vi "AutonTurning.vi"(7 "Re-Init":bool, 9 "SensorInputData":T1, 10 "arguments":string[](array[string]), 11 "HMI to Control":T2) -> (2 "SensorInputDataOut":T1, 3 "HMI to Control Out":T2, 4 "Done":bool)   [LabVIEW 2014]
uses:
  Typedefs/HMI_to_Control.ctl
  Typedefs/Arm States.ctl
  Typedefs/ClawStates.ctl
  Typedefs/IntakeWheelSenseOrManual.ctl
  Typedefs/SensorInputData.ctl
  scriptlib/auto_data.vi
panel:
  in  "Ernie kP":dbl=0.05 format="%#_13g"
  in  "?":cluster{"Yaw":dbl, "Setpoint":dbl}
  out "Yaw vs Setpoint Graph":cluster{"Yaw":dbl, "Setpoint":dbl}(graph)
  in  "InRangeTimer":i32=200
  in  "Permissable Error Range":dbl=3.0
  in  "kD":dbl=0.001
  in  "IntegralCap":dbl=0.1 format="%#_13g"
  in  "kI":dbl=0.001
  in  "Bert kP":dbl=0.05 format="%#_13g"
  # "Graphs the current value of the sensor for easy comparison to setpoint"
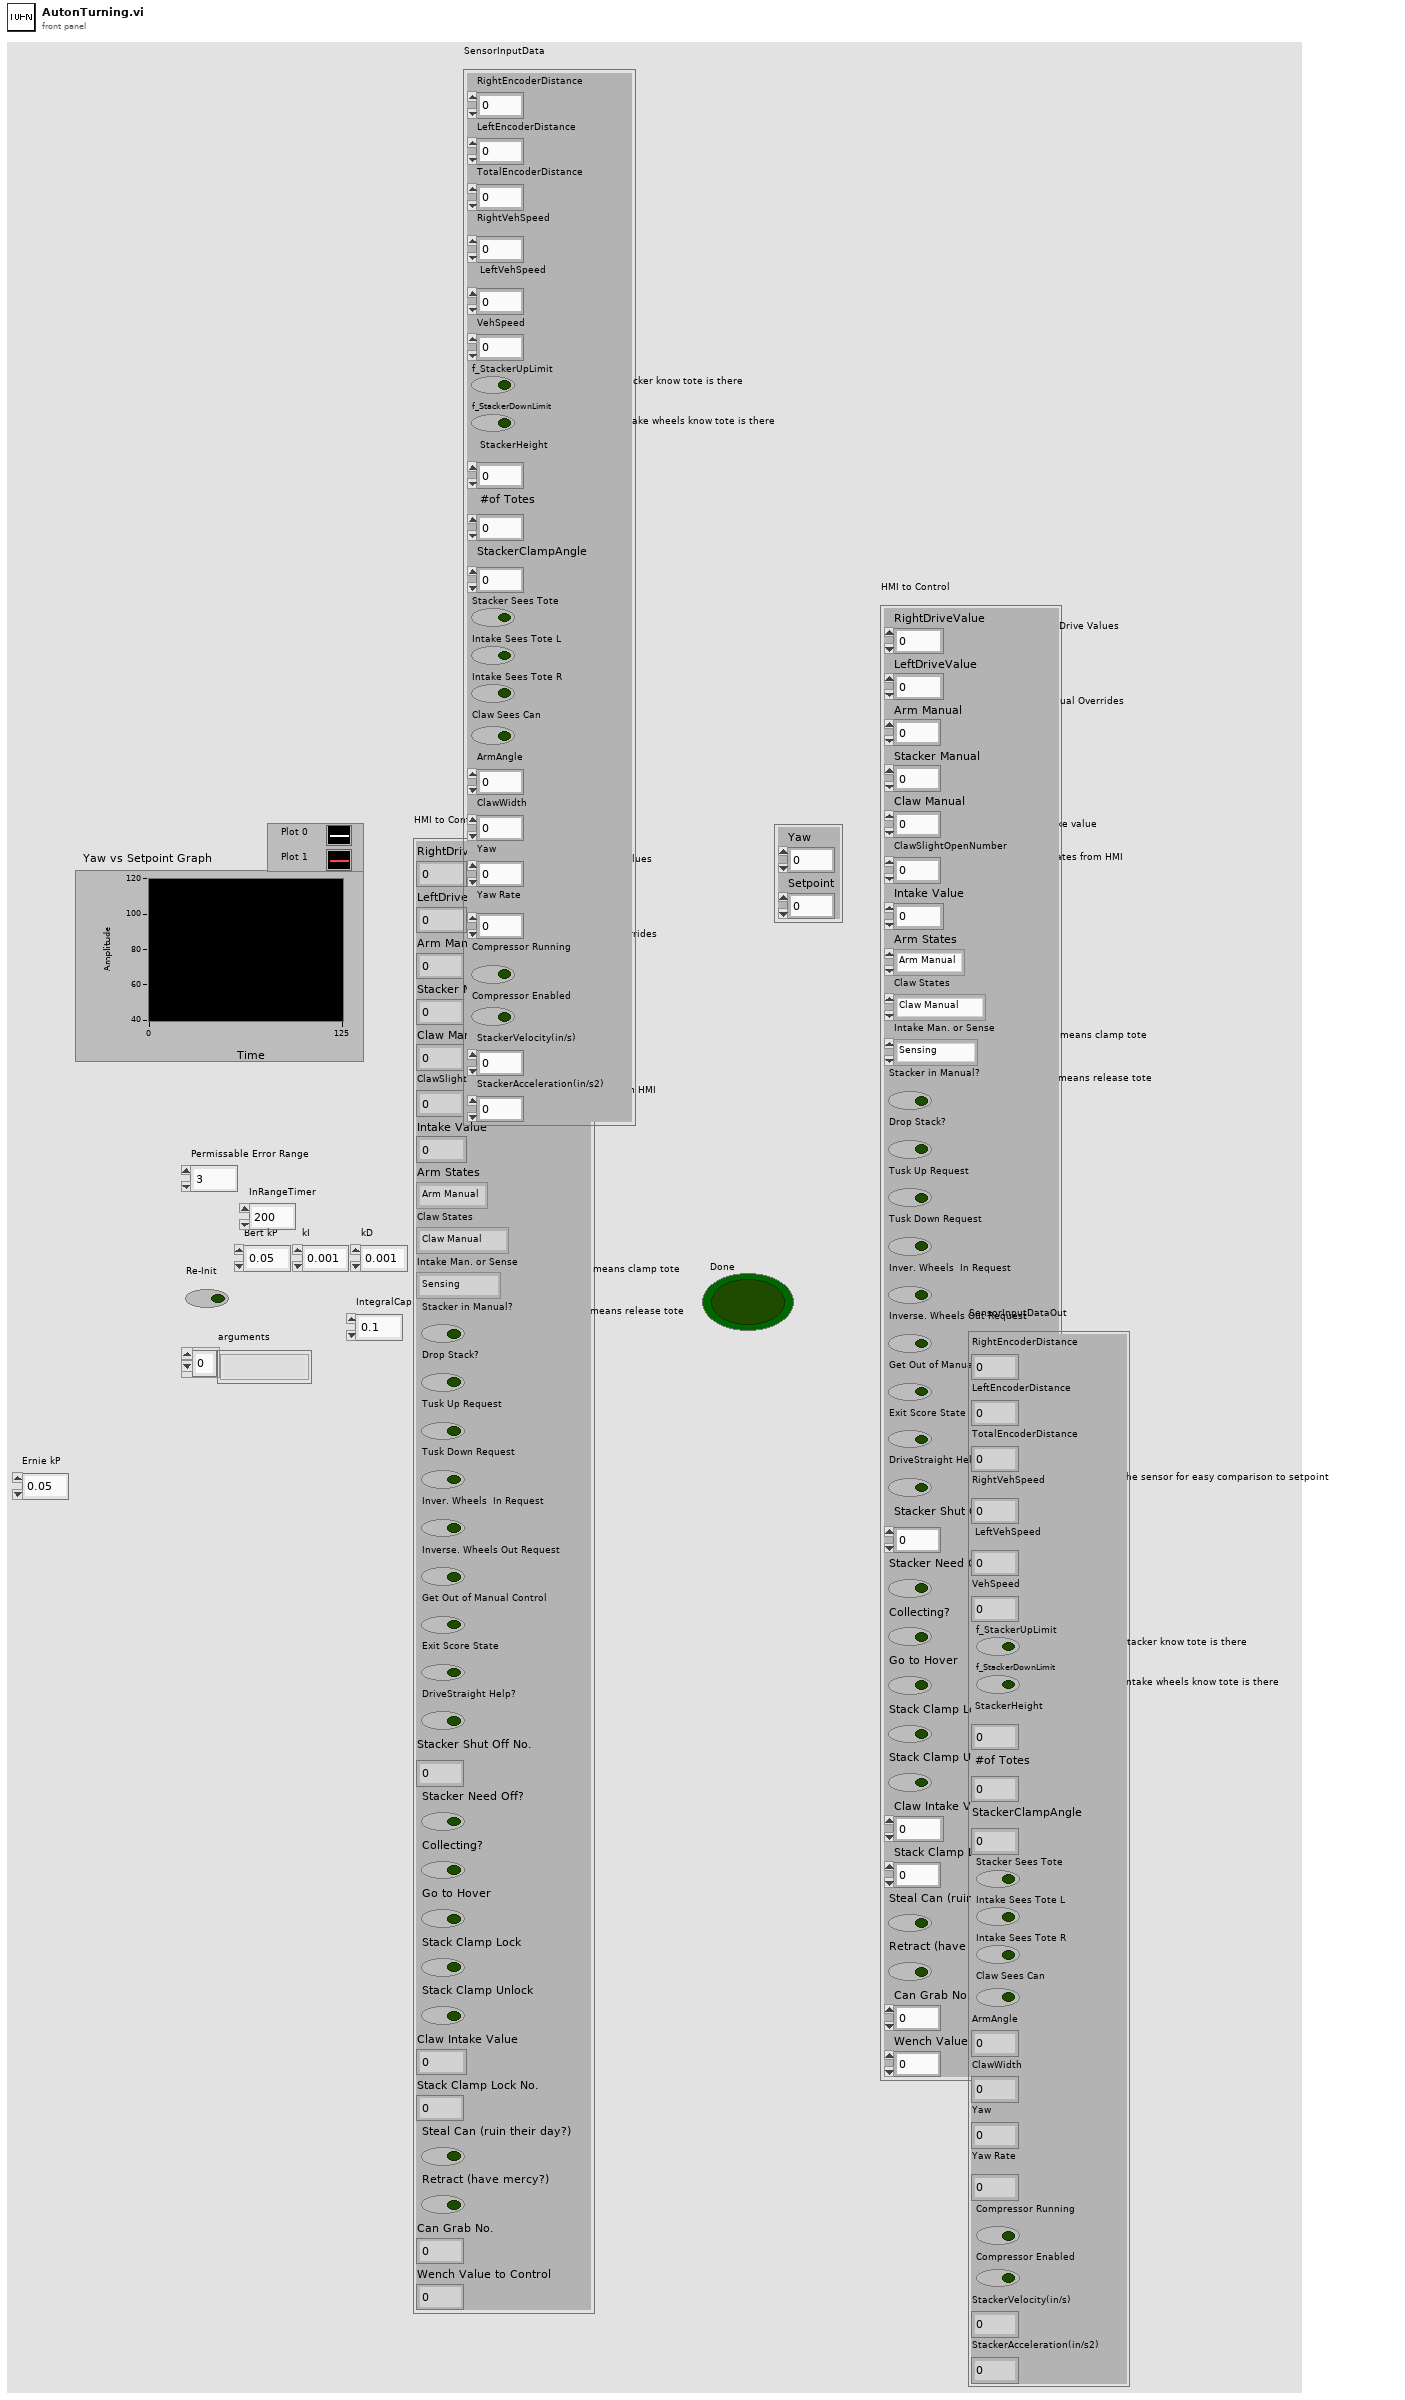
[diagram p1: front panel]
types:
  T1 = typedef "SensorInputData.ctl" = cluster{"RightEncoderDistance":dbl, "LeftEncoderDistance":dbl, "TotalEncoderDistance":dbl, "RightVehSpeed":dbl, "LeftVehSpeed":dbl, "VehSpeed":dbl, "f_StackerUpLimit":bool, "f_StackerDownLimit":bool, "StackerHeight":dbl, "#of Totes":u8, "StackerClampAngle":dbl, "Stacker Sees Tote":bool, "Intake Sees Tote L":bool, "Intake Sees Tote R":bool, "Claw Sees Can":bool, "ArmAngle":dbl, "ClawWidth":dbl, "Yaw":dbl, "Yaw Rate":dbl, "Compressor Running":bool, "Compressor Enabled":bool, "StackerVelocity(in/s)":dbl, "StackerAcceleration(in/s2)":dbl}
  T2 = typedef "HMI_to_Control.ctl" = cluster{"RightDriveValue":dbl, "LeftDriveValue":dbl, "Arm Manual ":dbl, "Stacker Manual ":dbl, "Claw Manual ":dbl, "ClawSlightOpenNumber":i8, "Intake Value ":sgl, "Arm States":T3, "Claw States":T4, "Intake Man. or Sense":T5, "Stacker in Manual?":bool, "Drop Stack? ":bool, "Tusk Up Request":bool, "Tusk Down Request":bool, "Inver. Wheels  In Request":bool, "Inverse. Wheels Out Request ":bool, "Get Out of Manual Control":bool, "Exit Score State":bool, "DriveStraight Help?":bool, "Stacker Shut Off No.":i8, "Stacker Need Off?":bool, "Collecting?":bool, "Go to Hover":bool, "Stack Clamp Lock ":bool, "Stack Clamp Unlock ":bool, "Claw Intake Value ":sgl, "Stack Clamp Lock No. ":i8, "Steal Can (ruin their day?)":bool, "Retract (have mercy?)":bool, "Can Grab No. ":i8, "Wench Value to Control ":dbl}
  T3 = typedef "Arm States.ctl" = enum16{"Arm Manual ", "Ground", "Step", "1 Tote", "2 Tote", "3 Tote", "4 Tote", "5 Tote", "6 Tote", "Flip Can Arm", "Grab Can in auto", "Nudge"}
  T4 = typedef "ClawStates.ctl" = enum16{"Claw Manual ", "Claw Open", "Claw Closed", "Claw Slight Open", "Flip Can"}
  T5 = typedef "IntakeWheelSenseOrManual.ctl" = enum16{"Sensing", "Manual "}
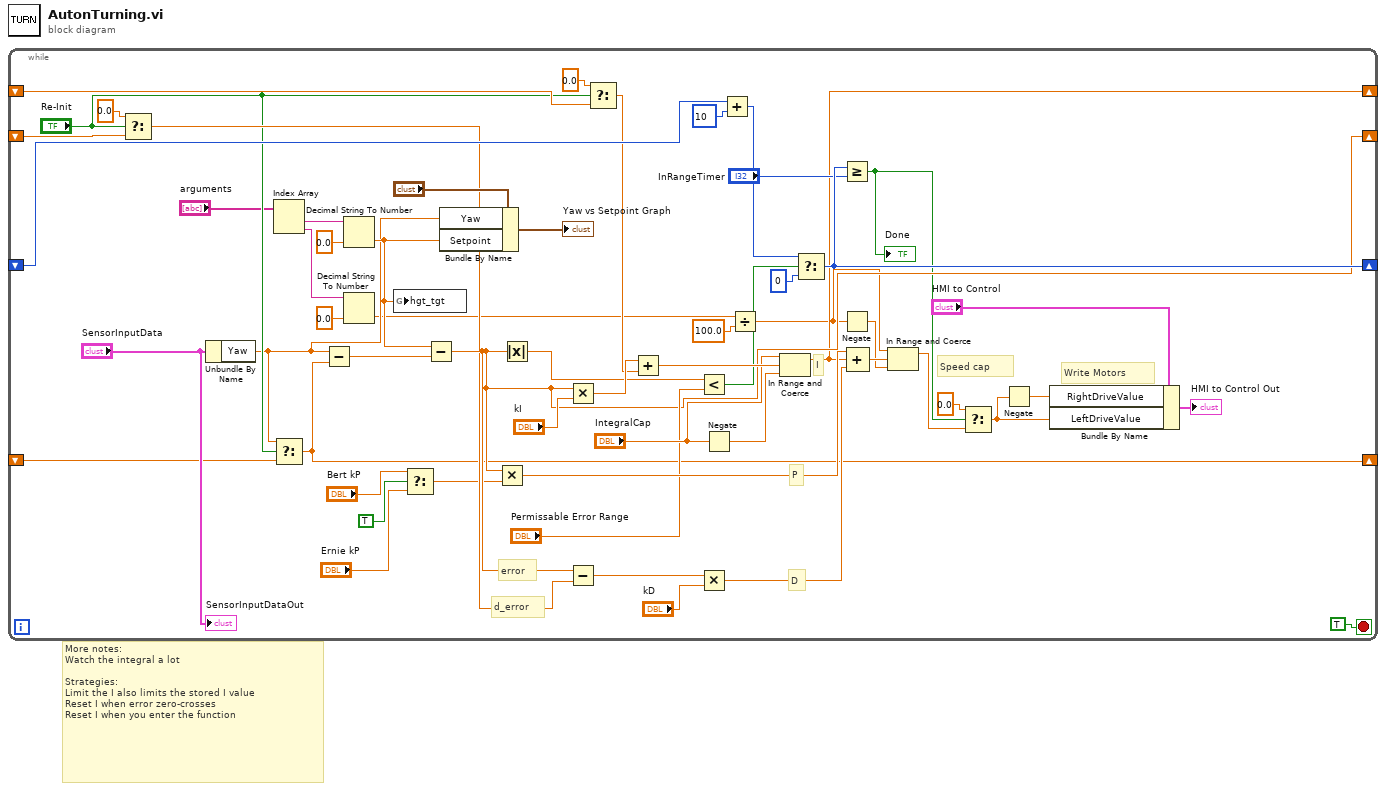
[diagram p0: block diagram]
diagram:
  # "More notes: \nWatch the integral a lot\n\nStrategies:\nLimit the I also limits the stored I value\nReset I when error zero-crosses\nReset I when you enter the function"
  n1 = while {
    shift-right: [w23] -> _
    shift-left: _ -> [w29]
    shift-right: [w35] -> _
    shift-left: _ -> [w26]
    shift-right: [w40] -> _
    shift-left: _ -> [w42]
    shift-right: [w11] -> _
    shift-left: _ -> [w12]
    stop <- TRUE stop-if-true
    # "I"
    # "Speed cap"
    # "Write Motors"
    # "D"
    # "d_error"
    # "error"
    # "P"
    n2 = Select(t=0.0, s="Re-Init", f=w26) -> (s? t:f=w25:dbl)
    n3 = Unbundle By Name("SensorInputData") -> ("Yaw"=w10:dbl)
    n4 = Index Array(array="arguments") -> (element #1=w14:string, element #2=w5:string)  [unwired: 2 in]
    n5 = Select(t=w10, s="Re-Init", f=w12) -> (s? t:f=w11:dbl)
    n6 = Subtract(x=w10, y=w11) -> (x-y=w16:dbl)
    n7 = Decimal String To Number(string=w14, default (0L)=0.0) -> (number=w17:dbl)  [unwired: 1 in, 1 out]
    n8 = Decimal String To Number(string=w5, default (0L)=0.0) -> (number=w2:dbl)  [unwired: 1 in, 1 out]
    n9 = global write "auto_data.vi" "hgt_tgt"(w17) -> ()
    n10 = Select(t="Bert kP", s=TRUE ("On Bert?"), f="Ernie kP") -> (s? t:f=w7:dbl)
    n11 = Subtract(x=w17, y=w16) -> (x-y=w35:dbl)
    n12 = Bundle By Name(cluster="?", "Yaw"=w10, "Setpoint"=w17) -> (→"Yaw vs Setpoint Graph":cluster{"Yaw":dbl, "Setpoint":dbl})
    n13 = Multiply(x=w35, y=w7) -> (x*y=w56:dbl)
    n14 = Absolute Value(x=w35) -> (abs(x)=w47:dbl)
    n15 = Multiply(x=w35, y="kI") -> (x*y=w54:dbl)
    n16 = Subtract(x=w35, y=w25) -> (x-y=w50:dbl)
    n17 = Select(t=0.0, s="Re-Init", f=w29) -> (s? t:f=w28:dbl)
    n18 = Add(x=w54, y=w28) -> (x+y=w53:dbl)
    n19 = Less?(x=w47, y="Permissable Error Range") -> (x < y?=w45:bool)
    n20 = Multiply(x=w50, y="kD") -> (x*y=w48:dbl)
    n21 = Negate(x="IntegralCap") -> (-x=w52:dbl)
    n22 = Add(x=w42, y=i8 10) -> (x+y=w41:i32)
    n23 = Divide(x=w2, y=100.0) -> (x/y=w1:dbl)
    n24 = In Range and Coerce(upper limit="IntegralCap", x=w53, lower limit=w52) -> (coerced(x)=w23:dbl)  [unwired: 1 out]
    n25 = Select(t=w41, s=w45, f=0 ("InRangeTimer 2")) -> (s? t:f=w40:i32)
    n26 = Greater Or Equal?(x=w40, y="InRangeTimer") -> (x >= y?=w20:bool)
    "Done" <- w20
    n27 = Negate(x=w1) -> (-x=w33:dbl)
    n28 = Compound Arithmetic op=ADD(w56, w23, w48) -> (w34:dbl)
    n29 = In Range and Coerce(upper limit=w1, x=w34, lower limit=w33) -> (coerced(x)=w22:dbl)  [unwired: 1 out]
    n30 = Select(t=0.0, s=w20, f=w22) -> (s? t:f=w21:dbl)
    n31 = Negate(x=w21) -> (-x=w30:dbl)
    n32 = Bundle By Name(cluster="HMI to Control", "RightDriveValue"=w30, "LeftDriveValue"=w21) -> (→"HMI to Control Out":T2)
    "SensorInputDataOut" <- "SensorInputData"
  }
